vi "Measure Statistics.vi"(6 "Measurement":T1, 8 "error in (no error)":errorcluster, 9 "No. Reads":i32=2000, 10 "Channel":T3, 11 "MSOX6004 in":refnum<class "MSOX6004.lvclass">) -> (0 "error out":errorcluster, 2 "Statistics":T2, 3 "MSOX6004 out":refnum<class "MSOX6004.lvclass">)   [LabVIEW 2018, in "MSOX6004.lvlib" / "MSOX6004.lvclass"]
uses:
  MSOX6004.lvclass
  PPLs/Oscilloscope/Parent/Oscilloscope.lvlibp/Custom Controls/Analog Channels.ctl
  PPLs/Oscilloscope/Parent/Oscilloscope.lvlibp/Custom Controls/Measurement.ctl
  MSOX6004.lvclass/MSOX6004.ctl
  <instrlib>/Keysight InfiniiVision/Keysight InfiniiVision.lvlib
  PPLs/Oscilloscope/Parent/Oscilloscope.lvlibp
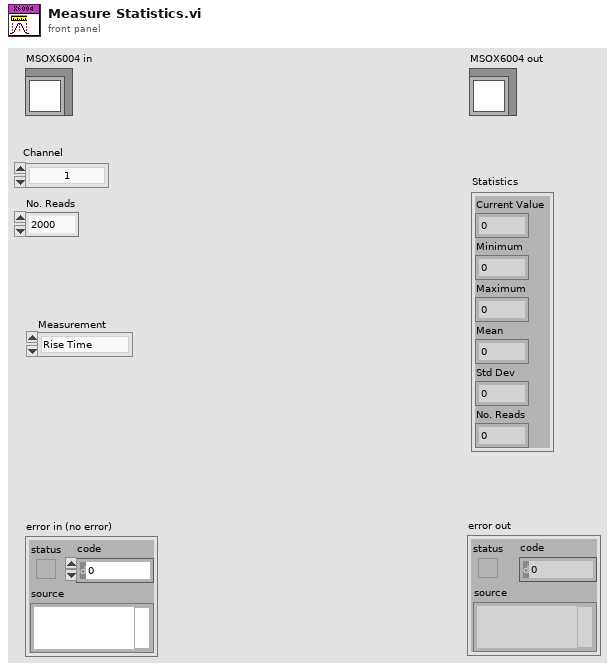
[diagram p1: front panel]
types:
  T1 = typedef "Oscilloscope.lvlibp/Measurement.ctl" = enum16{"Rise Time", "Fall Time", "Frequency", "Period", "RMS (V)", "Peak-Peak (V)", "Max (V)", "Min (V)", "High State (V)", "Low State (V)", "Average (V)", "Width (Negative)", "Width (Positive)", "Duty Cycle (Negative)", "Duty Cycle (Positive)", "Amplitude", "Cycle RMS (V)", "Cycle Avg (V)", "Overshoot", "Preshoot", "Time at Max", "Frequency Counter", "Time at Min", "Delay", "Value at Time", "Phase", "Time at Value", "Time of Edge", "Area", "Burst Width", "Falling Edge Count", "Rising Edge Count", "Falling Pulse Count", "Rising Pulse Count", "Std Dev", "Pulse Width"}
  T2 = cluster{"Current Value":dbl, "Minimum":dbl, "Maximum":dbl, "Mean":dbl, "Std Dev":dbl, "No. Reads":dbl}
  T3 = typedef "Oscilloscope.lvlibp/Analog Channels.ctl" = enum16{"1", "2", "3", "4", "5", "6", "7", "8", "9", "10", "11", "12", "13", "14", "15", "16"}
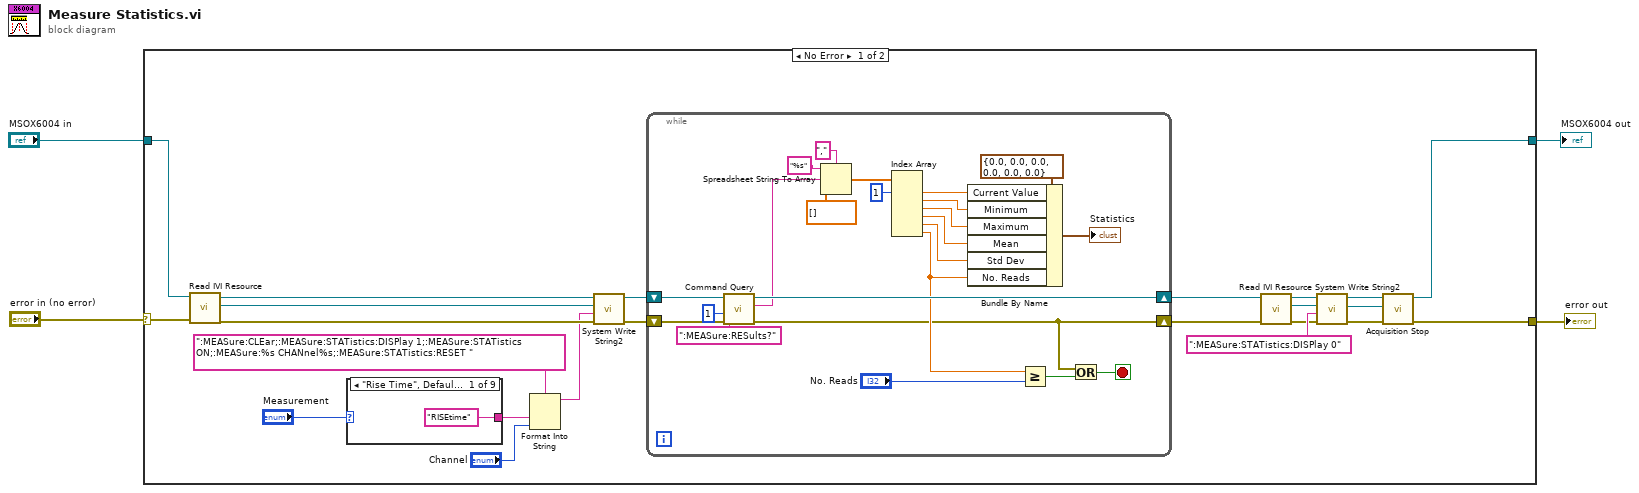
[diagram p0: block diagram]
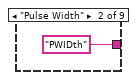
[diagram p2: hidden frame]
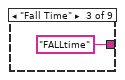
[diagram p3: hidden frame]
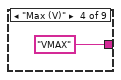
[diagram p4: hidden frame]
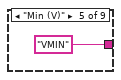
[diagram p5: hidden frame]
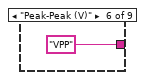
[diagram p6: hidden frame]
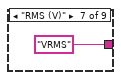
[diagram p7: hidden frame]
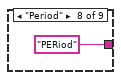
[diagram p8: hidden frame]
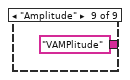
[diagram p9: hidden frame]
diagram:
  n1 = case shown="No Error" "error in (no error)" {
    selector: "error in (no error)" -> [w24 w57]
    tunnel: "MSOX6004 in" -> [w23 w58]
    tunnel: [w10 w58] -> w2
    tunnel: [w5 w57] -> w1
    frame No Error {
      n2 = call "Read IVI Resource.vi"("error in (no error)"=w24, "MSOX6004 in"=w23) -> ("error out"=w21:errorcluster, "IVI Resource"=w22:refnum<k15>, "MSOX6004 out"=w18:refnum<class "MSOX6004.lvclass">)  [unwired: 7 in]
      n3 = case shown="\"Rise Time\", Default" "Measurement" {
        tunnel: ["RISEtime" "PWIDth" "FALLtime" "VMAX" "VMIN" "VPP" "VRMS" "PERiod" "VAMPlitude"] -> w15
        frame "Rise Time", Default {
        }
        frame "Pulse Width" {
        }
        frame "Fall Time" {
        }
        frame "Max (V)" {
        }
        frame "Min (V)" {
        }
        frame "Peak-Peak (V)" {
        }
        frame "RMS (V)" {
        }
        frame "Period" {
        }
        frame "Amplitude" {
        }
      }
      n4 = Format Into String(format string=":MEASure:CLEar;:MEASure:STATistics:DISPlay 1;:MEASure:STATistics ON;:MEASure:%s CHANnel%s;:MEASure:STATistics:RESET ", w15, "Channel") -> (resulting string=w19:string)  [unwired: 2 in, 1 out]
      n5 = call <instrlib>:"System Write String2.vi"("error in (no error)"=w21, "Data"=w19, "instrument handle"=w22) -> ("error out"=w17:errorcluster)  [unwired: 7 in, 1 out]
      n6 = while {
        shift-right: [w45] -> w11
        shift-left: w18 -> [w47]
        shift-right: [w28] -> w13
        shift-left: w17 -> [w46]
        stop <- w26 stop-if-true
        n7 = call "Command Query.vi"("error in (no error)"=w46, "Delay (ms)"=u32 1, "Command"=":MEASure:RESults?", "MSOX6004 in"=w47) -> ("error out"=w28:errorcluster, "Response"=w33:string, "MSOX6004 out"=w45:refnum<class "MSOX6004.lvclass">)  [unwired: 5 in]
        n8 = Spreadsheet String To Array(delimiter (Tab)=",", format string="%s", spreadsheet string=w33, array type (2D Dbl)=dbl[] []) -> (array=w41:dbl[])
        n9 = Index Array(array=w41, index #1=1 ("index")) -> (element #1=w38:dbl, element #2=w37:dbl, element #3=w36:dbl, element #4=w35:dbl, element #5=w34:dbl, element #6=w29:dbl)  [unwired: 5 in]
        n10 = Bundle By Name(cluster=T2 {"Current Value"=0.0, "Minimum"=0.0, "Maximum"=0.0, "Mean"=0.0, "Std Dev"=0.0, "No. Reads"=0.0} ("Statistics"), "Current Value"=w38, "Minimum"=w37, "Maximum"=w36, "Mean"=w35, "Std Dev"=w34, "No. Reads"=w29) -> (→"Statistics":T2)
        n11 = Greater Or Equal?(x=w29, y="No. Reads") -> (x >= y?=w27:bool)
        n12 = Or(x=w28, y=w27) -> (x .or. y?=w26:bool)
      }
      n13 = call "Read IVI Resource.vi"("error in (no error)"=w13, "MSOX6004 in"=w11) -> ("error out"=w7:errorcluster, "IVI Resource"=w12:refnum<k15>, "MSOX6004 out"=w10:refnum<class "MSOX6004.lvclass">)  [unwired: 7 in]
      n14 = call <instrlib>:"System Write String2.vi"("error in (no error)"=w7, "Data"=":MEASure:STATistics:DISPlay 0", "instrument handle"=w12) -> ("error out"=w6:errorcluster, "instrument handle out"=w8:refnum<k15>)  [unwired: 7 in]
      n15 = call <instrlib>:"Acquisition Stop.vi"("error in (no error)"=w6, "instrument handle"=w8) -> ("error out"=w5:errorcluster)  [unwired: 8 in, 1 out]
    }
    frame Error {
    }
  }
  "error out" <- w1
  "MSOX6004 out" <- w2
